vi "TestCode.vi"() -> ()   [LabVIEW 2019]
uses:
  D:/Personal/Blogs/Session Sharing/CS Code/SupplyTest/bin/Debug/TestProgram.SupplyTest.dll
  CS Code/SupplyTest/bin/Debug/TestProgram.SupplyTest.dll
panel:
  in  "Supplt Resource Name":refnum<k15>="VccSupply"
  in  "Stress Voltage Level":dbl=1.3 format="%#_13g"
  out "StressCurrent":dbl[](array[numeric])
  out "Source:DC Voltage:Voltage Level":dbl
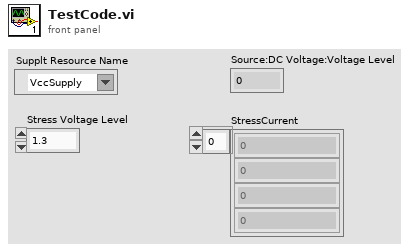
[diagram p1: front panel]
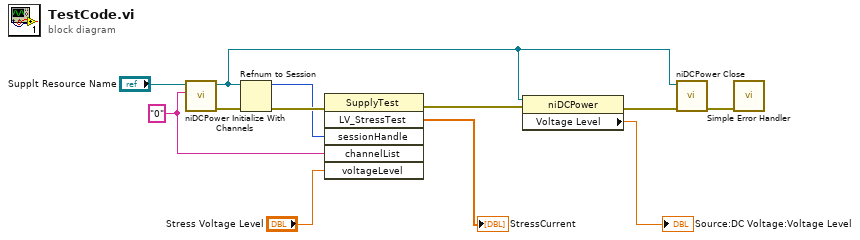
[diagram p0: block diagram]
diagram:
  w4 = "0" ("channels")
  n1 = call <instrlib>:"niDCPower Initialize With Channels.vi"("channels"=w4, "resource name"="Supplt Resource Name") -> ("error out"=w12:errorcluster, "instrument handle out"=w9:refnum<k15>)  [unwired: 8 in]
  n2 = Refnum to Session(4:w12, 7:w9) -> (0:w7:errorcluster, 3:w5:u64)
  n3 = invoke class="SupplyTest" method="LV_StressTest"(error in=w7, "sessionHandle"=w5, "channelList"=w4, "voltageLevel"="Stress Voltage Level") -> (error out=w6:errorcluster, "LV_StressTest"=→"StressCurrent":dbl[])  [unwired: 2 in, 4 out]
  n4 = property class="niDCPower"(reference=w9, error in=w6) -> (error out=w10:errorcluster, "Voltage Level"=→"Source:DC Voltage:Voltage Level":dbl)  [unwired: 1 out]
  n5 = call <instrlib>:"niDCPower Close.vi"("error in (no error)"=w10, "instrument handle"=w9) -> ("error out"=w1:errorcluster)  [unwired: 9 in]
  n6 = call <vilib>:"Simple Error Handler.vi"("error in (no error)"=w1) -> ()  [unwired: 4 in, 5 out]
